vi "FTW-Time-Remaining.vi"(0 "Total Work Units":i64, 5 "Work Units Complete":i64, 7 "Initial Timestamp":u32, 9 "Current Timestamp":u32, 11 "Window Size (for smoothing)":i32=15) -> (4 "Percent Done (0.0-100.0%)":dbl, 6 "Time Elapsed (msec)":u32, 8 "Estimated Time Remaining (msec)":u32, 10 "Current Rate (Units of Work per sec)":dbl, 15 "Settled?":bool)   [LabVIEW 2013]
panel:
  # "Inputs"
  # "Outputs"
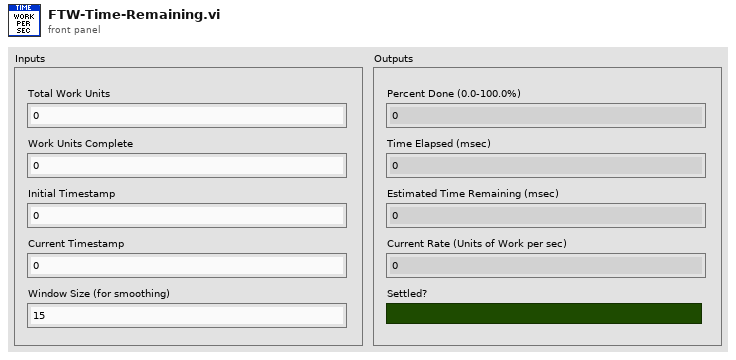
[diagram p1: front panel]
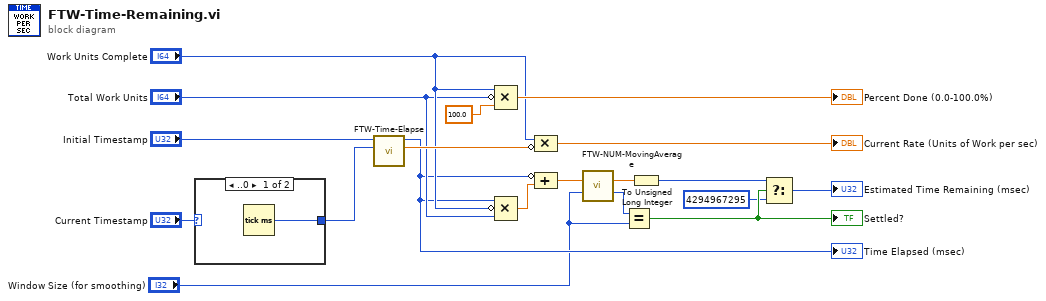
[diagram p0: block diagram]
diagram:
  n1 = case shown="..0" "Current Timestamp" {
    selector: "Current Timestamp" -> [_ w21]
    tunnel: [w20 w21] -> w10
    frame ..0 {
      n2 = Tick Count (ms)() -> (millisecond timer value=w20:u32)
    }
    frame Default {
    }
  }
  n3 = call "FTW-Time-Elapse.vi"("End Time"=w10, "Initial Time"="Initial Timestamp") -> ("Elapsed sec"=w16:dbl, "Elapsed msec"=w9:u32)  [unwired: 8 in]
  "Time Elapsed (msec)" <- w9
  n4 = Compound Arithmetic op=MULTIPLY("Work Units Complete", invert "Total Work Units", 100.0 ("value")) -> (→"Percent Done (0.0-100.0%)":dbl)
  n5 = Compound Arithmetic op=MULTIPLY(w9, invert "Work Units Complete", "Total Work Units") -> (w19:dbl)
  n6 = Compound Arithmetic op=MULTIPLY("Work Units Complete", invert w16) -> (→"Current Rate (Units of Work per sec)":dbl)
  n7 = Compound Arithmetic op=ADD(invert w9, w19) -> (w8:dbl)
  n8 = call "FTW-NUM-MovingAverage.vi"("New Value"=w8, "Window Size"="Window Size (for smoothing)") -> ("Average Value"=w4:dbl, "Items in Window"=w7:i32)  [unwired: 11 in, 1 out]
  n9 = Equal?(x=w7, y="Window Size (for smoothing)") -> (x = y?=w5:bool)
  "Settled?" <- w5
  n10 = To Unsigned Long Integer(number=w4) -> (unsigned 32bit integer=w1:u32)
  n11 = Select(t=w1, s=w5, f=u32 4294967295) -> (s? t:f=→"Estimated Time Remaining (msec)":u32)
